vi "Enable Disable.vi"(0 "Control/IndicatorRefnum":refnum<vi>[](array[refnum]), 5 "Boolean":bool, 11 "error in (no error)":errorcluster) -> (15 "error out":errorcluster)   [LabVIEW 2021, in "CustomSortPath.lvlib"]
doc: "Gets the control/indicator reference and boolean as input.Disables when boolean is false and enables when it is true."
uses:
  CustomSortPath.lvlib
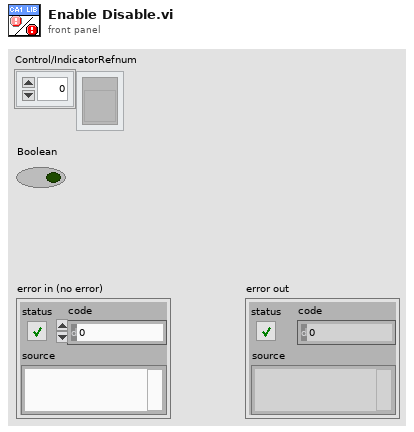
[diagram p1: front panel]
types:
  T1 = enum8{"Enabled", "Disabled", "Disabled and Grayed Out"}
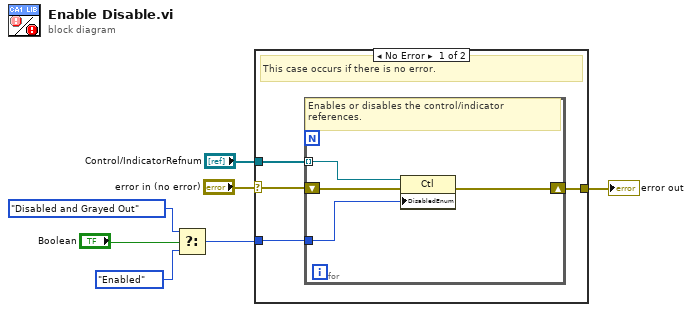
[diagram p0: block diagram]
diagram:
  n1 = Select(t=T1."Disabled and Grayed Out" ("Disabled"), s="Boolean", f=T1."Enabled" ("Disabled")) -> (s? t:f=w4:T1)
  n2 = case shown="No Error" "error in (no error)" {
    selector: "error in (no error)" -> [w9 w16]
    tunnel: w4 -> [w11 _]
    tunnel: "Control/IndicatorRefnum" -> [w10 _]
    tunnel: [w8 w16] -> w1
    frame No Error {
      # "This case occurs if there is no error."
      n3 = for {
        tunnel: w11 -> [w12]
        tunnel: w10 -> [w13] mode=indexing
        shift-right: [w14] -> w8
        shift-left: w9 -> [w15]
        # "Enables or disables the control/indicator references."
        n4 = property class="Ctl"(reference=w13, error in=w15, "DisabledEnum"=w12) -> (error out=w14:errorcluster)  [unwired: 1 out]
      }
    }
    frame Error {
      # "This case occurs if there is any error."
    }
  }
  "error out" <- w1
